vi "t2ns.vi"(1 "t/div":T1(ring)) -> (0 "ns/div":u32)   [LabVIEW 2009]
panel:
  # "=>"
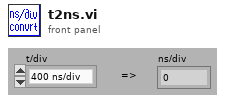
[diagram p1: front panel]
types:
  T1 = enum16{"400 ns/div", "1 us/div", "2 us/div", "4 us/div", "10 us/div", "20 us/div"}
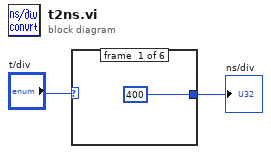
[diagram p0: block diagram]
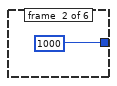
[diagram p2: hidden frame]
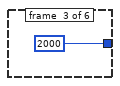
[diagram p3: hidden frame]
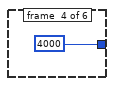
[diagram p4: hidden frame]
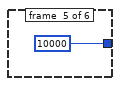
[diagram p5: hidden frame]
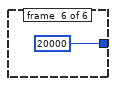
[diagram p6: hidden frame]
diagram:
  n1 = case shown="\"1 us/div\"" "t/div" {
    tunnel: [400 1000 2000 4000 10000 20000] -> w1
    frame #0 {
    }
    frame #1 {
    }
    frame #2 {
    }
    frame #3 {
    }
    frame #4 {
    }
    frame #5 {
    }
  }
  "ns/div" <- w1
